vi "Connect.vi"(8 "error in (no error)":errorcluster, 10 "Connection String":string, 11 "SqliteConnection in":refnum<class "DBC.lvclass">) -> (0 "error out":errorcluster, 3 "SqliteConnection out":refnum<class "DBC.lvclass">)   [LabVIEW 2020, in "ORM_DBC_Sqlite.lvlib" / "DBC.lvclass"]
uses:
  DBC.lvclass
  C:/Program Files/National Instruments/LabVIEW 2024/vi.lib/Viviota/shared/ORM_DBC_dotNet.lvlibp/dbcDotNet/ORM_DBC_dotNet.lvclass
  C:/Program Files/National Instruments/LabVIEW 2024/vi.lib/Viviota/shared/ORM.lvlibp/ORM/DbConnection/DbConnection.lvclass
  DBC.lvclass/DBC.ctl
  <vilib>/Viviota/shared/ORM_DBC_dotNet.lvlibp/dbcDotNet/Write connection.vi
  <vilib>/Viviota/shared/ORM.lvlibp/ORM/DbConnection/Write ColumnNameEqualsValueFormat.vi
  <vilib>/Viviota/shared/ORM.lvlibp/ORM/DbConnection/Write ColumnNameFormat.vi
  <vilib>/Viviota/shared/ORM.lvlibp/ORM/DbConnection/Write LastIdentityQuery.vi
  <vilib>/Viviota/shared/ORM.lvlibp/ORM/DbConnection/Write TableNameFormat.vi
  C:/Viviota/Projects/R&D/__OpenSource/VIV_ORM/libraries/sqlite/System.Data.SQLite.dll
  libraries/sqlite/System.Data.SQLite.dll
  <vilib>/regexp/Match Regular Expression.xnode
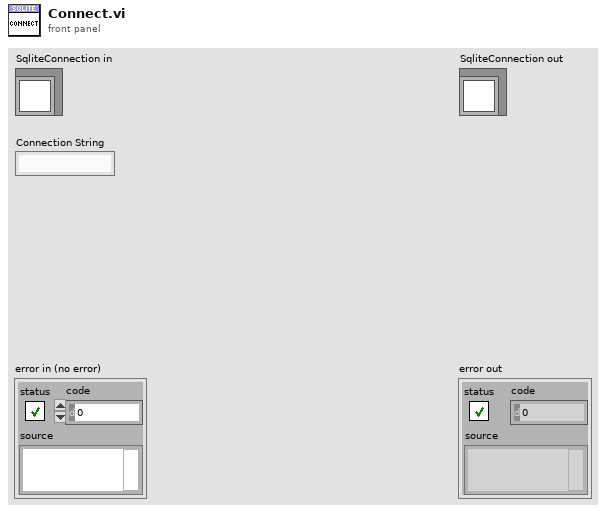
[diagram p1: front panel]
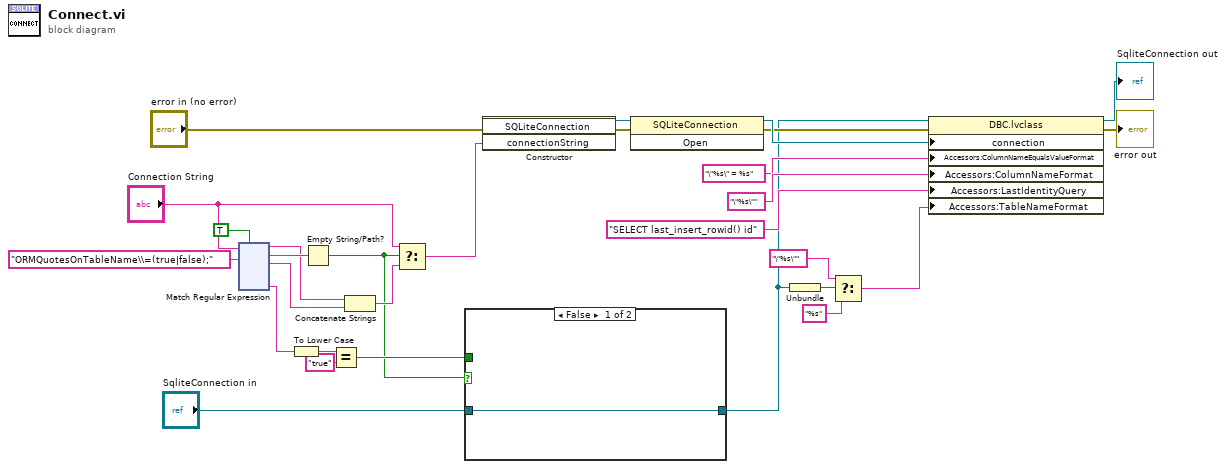
[diagram p0: block diagram]
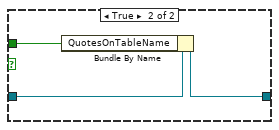
[diagram p2: hidden frame]
diagram:
  n1 = xnode "Match Regular Expression"("input string"="Connection String", "regular expression"="ORMQuotesOnTableName\\=(true|false);", "ignore case? (F)"=TRUE) -> ("before match"=w11:string, "whole match"=w12:string, "after match"=w10:string, "submatch 1"=w6:string)  [unwired: 3 in, 2 out]
  n2 = To Lower Case(string=w6) -> (all lower case string=w5:string)
  n3 = Empty String/Path?(string/path=w12) -> (empty?=w1:bool)
  n4 = Equal?(x=w5, y="true") -> (x = y?=w2:bool)
  n5 = Concatenate Strings(w11, w10) -> (w8:string)
  n6 = Select(t="Connection String", s=w1, f=w8) -> (s? t:f=w7:string)
  n7 = case shown="False" w1 {
    tunnel: "SqliteConnection in" -> [w30 w33]
    tunnel: [w30 w32] -> w3
    tunnel: w2 -> [_ w31]
    frame False {
    }
    frame True {
      n8 = Bundle By Name(cluster=w33, "QuotesOnTableName"=w31) -> (w32:refnum<class "DBC.lvclass">)
    }
  }
  n9 = constructor class="SQLiteConnection"(error in="error in (no error)", "connectionString"=w7) -> (reference out=w29:refnum<k24>, error out=w27:errorcluster)  [unwired: 2 in, 2 out]
  n10 = invoke class="SQLiteConnection" method="Open"(reference=w29, error in=w27) -> (reference out=w26:refnum<k24>, error out=w20:errorcluster)  [unwired: 1 in, 1 out]
  n11 = Unbundle(w3) -> (w18:bool)
  n12 = Select(t="\"%s\"" ("TableNameFormat"), s=w18, f="%s" ("TableNameFormat")) -> (s? t:f=w15:string)
  n13 = property class="DBC.lvclass"(reference=w3, error in=w20, "connection"=w26, "Accessors:ColumnNameEqualsValueFormat"="\"%s\" = %s" ("ColumnNameFormat"), "Accessors:ColumnNameFormat"="\"%s\"" ("ColumnNameFormat"), "Accessors:LastIdentityQuery"="SELECT last_insert_rowid() id" ("LastIdentityQuery"), "Accessors:TableNameFormat"=w15) -> (reference out=→"SqliteConnection out":refnum<class "DBC.lvclass">, error out=→"error out":errorcluster)
